vi "Dane_wej.vi"(11 "file path (use dialog)":path=path "F:/SUS/SUS_Lab/chka_F_Pg30.txt") -> (1 "L/min":dbl, 2 "Twe":dbl, 3 "Moc grzałki":dbl)   [LabVIEW 2020]
uses:
  <vilib>/Utility/file.llb/Read From Spreadsheet File (DBL).vi
panel:
  out "all rows":dbl[][](array[numeric]) format="%0.3f"
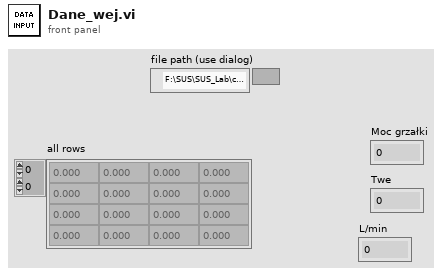
[diagram p1: front panel]
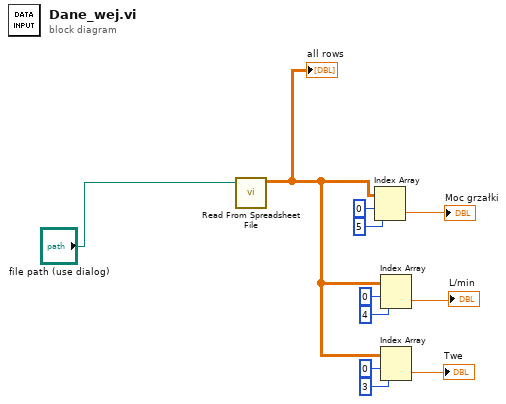
[diagram p0: block diagram]
diagram:
  n1 = call-poly <vilib>:"Read From Spreadsheet File.vi"("file path (dialog if empty)"="file path (use dialog)") -> ("all rows"=w5:dbl[][])  [unwired: 6 in, 4 out]
  "all rows" <- w5
  n2 = Index Array(array=w5, index (row)=0, index (col)=5 ("disabled index (col)")) -> (element=→"Moc grzałki":dbl)
  n3 = Index Array(array=w5, index (row)=0, index (col)=4 ("disabled index (col)")) -> (element=→"L/min":dbl)
  n4 = Index Array(array=w5, index (row)=0, index (col)=3 ("disabled index (col)")) -> (element=→"Twe":dbl)
